vi "Create Message CSV.vi"(8 "Error In":errorcluster, 11 "Message":T1) -> (0 "Error Out":errorcluster, 3 "CSV":string)   [LabVIEW 2014, in "LV-Logger.lvlib"]
uses:
  LV-Logger.lvlib
  Controls/Message.ctl
  Controls/Tag.ctl
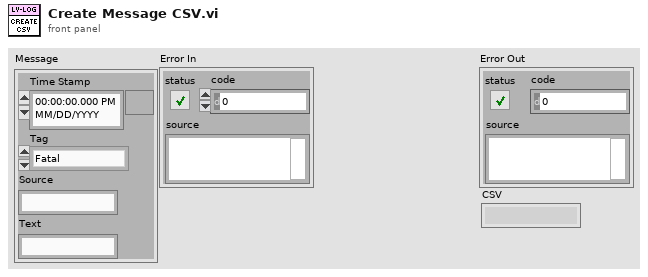
[diagram p1: front panel]
types:
  T1 = typedef "LV-Logger.lvlib/Message.ctl" = cluster{"Time Stamp":timestamp, "Tag":T2, "Source":string, "Text":string}
  T2 = typedef "LV-Logger.lvlib/Tag.ctl" = enum16{"Fatal", "Error", "Warn", "Info", "Debug", "Trace"}
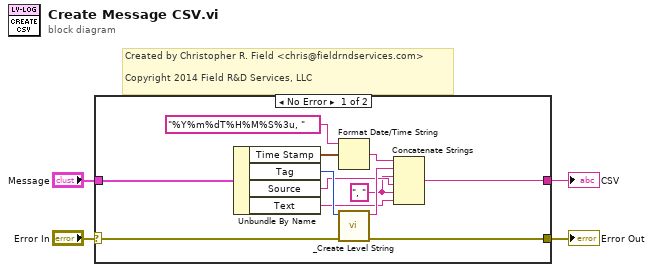
[diagram p0: block diagram]
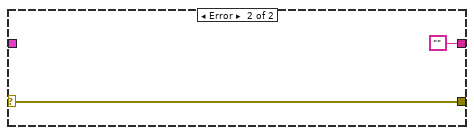
[diagram p2: hidden frame]
diagram:
  # "Created by Christopher R. Field <chris@fieldrndservices.com>\n\nCopyright 2014 Field R&D Services, LLC"
  n1 = case shown="No Error" "Error In" {
    selector: "Error In" -> [w12 w18]
    tunnel: "Message" -> [w16 _]
    tunnel: [w6 w18] -> w2
    tunnel: [w5 ""] -> w1
    frame No Error {
      w8 = ", " ("string")
      n2 = Unbundle By Name(w16) -> ("Time Stamp"=w15:timestamp, "Tag"=w13:T2, "Source"=w9:string, "Text"=w7:string)
      n3 = Format Date/Time String(time format string (%c)="%Y%m%dT%H%M%S%3u, ", seconds (now)=w15) -> (date/time string=w11:string)  [unwired: 1 in]
      n4 = call "_Create Level String.vi"("Error In"=w12, "Level"=w13) -> ("Error Out"=w6:errorcluster, "String"=w10:string)  [unwired: 8 in]
      n5 = Concatenate Strings(w11, w10, w8, w9, w8, w7) -> (w5:string)
    }
    frame Error {
    }
  }
  "Error Out" <- w2
  "CSV" <- w1
